vi "Pack for gRPC.vi"(8 "error in":errorcluster, 9 "configuration / results":enum16{"Configuration", "Results"}(ring), 10 "data value":variant, 11 "measurement plugin in":refnum<class "FPT_Compression.lvclass">) -> (0 "error out":errorcluster, 2 "any":T1, 3 "measurement plugin out":refnum<class "FPT_Compression.lvclass">)   [LabVIEW 2023, in "FPT_Compression.lvclass"]
uses:
  FPT_Compression.lvclass
  <vilib>/gRPC/LabVIEW gRPC Library/Shared/Any.ctl
  C:/Program Files/National Instruments/LabVIEW 2023/vi.lib/Plug-In SDKs/Measurements/Measurement Plugin Service/Measurement Plugin Service.lvclass
  Measurement Configuration.ctl
  Measurement Results.ctl
  2eca732d-dbaa-43bf-a7dd-ede2da65bc1b.vi
  a6012965-5700-4384-8228-972e71b6560c.vi
  <vilib>/gRPC/LabVIEW gRPC Library/Server API/Translate Protobuf Error.vi
  <vilib>/AdvancedString/1D String Array to Delimited String.vi
  <vilib>/gRPC/LabVIEW gRPC Library/Server API/Server/Get Server DLL Path.vi
  <vilib>/Plug-In SDKs/Measurements/Measurement Plugin Service/Measurement Plugin Service.lvclass
  <vilib>/gRPC/LabVIEW gRPC Library/grpc-lvsupport-release.lvlib
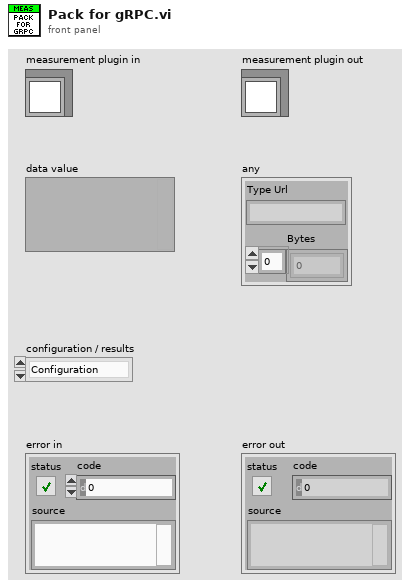
[diagram p1: front panel]
types:
  T1 = typedef "grpc-lvsupport-release.lvlib/Any.ctl" = cluster{"Type Url":string, "Bytes":u8[]}
  T2 = typedef "grpc-lvsupport-release.lvlib/grpcId.ctl" = u64
  T3 = typedef "FPT_Compression.lvclass/Measurement Configuration.ctl" = cluster{"Automation Test":bool, "Power sequencing file path":string, "SMU name":string, "SMU channel":string, "RFSG name":string, "RFSG port":string, "RFSG attenuation mode":enum32{"<None>", "Constant Attenuation", "s2p File"}, "RFSG external attenuation (dB)":dbl, "RFSG s-parameters orientation":enum32{"Port1 Towards DUT", "Port2 Towards DUT"}, "RFSG s2p file path":string, "RFmx name":string, "RFmx port":string, "RFmx attenuation mode":enum32{"<None>", "Constant Attenuation", "s2p File"}, "RFmx external attenuation (dB)":dbl, "RFmx attenuation path name":string, "RFmx s-parameters orientation":enum32{"Port1 Towards DUT", "Port2 Towards DUT"}, "RFmx attenuation s2p path name":string, "RFmx s2p file path":string, "Compression_Expected DUT Gain (dB)":dbl, "Compression_Max Linear Range (dBm)":dbl, "Compression_Compression Point (dB)":dbl, "Compression_Target Pin (dBm)":dbl, "Compression_RFSG Frequency Start (Hz)":dbl, "Compression_RFSG Frequency Stop (Hz)":dbl, "Compression_RFSG Number of Frequency Step":i32, "Compression_RFSG Power Start (dBm)":dbl, "Compression_RFSG Power Stop(dBm)":dbl, "Compression_RFSG Power Step Size (dB)":dbl, "Compression_RBW (Hz)":dbl, "Compression_RF Measurement Interval (s)":dbl, "Compression_DC Measurement Interval (s)":dbl, "Compression_Stimulus Mode":enum32{"Constant Power and RF", "Constant Power and Pulsed RF", "Pulsed Power and RF"}, "CP_CW_DC Source Delay (s)":dbl, "CP_PRF_DC Source Delay (s)":dbl, "CP_PRF_RFmx Trigger Delay (s)":dbl, "CP_PRF_RF Pulse Width (s)":dbl, "CP_PRF_PRI (s)":dbl, "PP_PRF_DC Source Delay (s)":dbl, "PP_PRF_RFmx Trigger Delay (s)":dbl, "PP_PRF_RF Pulse Width (s)":dbl, "PP_PRF_PRI (s)":dbl, "PP_PRF_DC Pulse Width (s)":dbl, "PP_PRF_ON Current Limit (A)":dbl, "PP_PRF_Bias Voltage Level (V)":dbl, "PP_PRF_Bias Current Limit (A)":dbl, "Power sequencing file validity check":bool}
  T4 = typedef "FPT_Compression.lvclass/Measurement Results.ctl" = cluster{"Status":string, "per Freq Plot Names":string[], "Linear Gain vs Freq":dbl[][], "OPxdB vs Freq":dbl[][], "Pout@Pin vs Freq":dbl[][], "Gain@Pin vs Freq":dbl[][], "PAE@Pin vs Freq":dbl[][], "Pout vs Pin per Freq":dbl[][], "Gain vs Pin per Freq":dbl[][], "PAE vs Pin per Freq":dbl[][], "Pout@Pin (Mean)":dbl, "Gain@Pin (Mean)":dbl, "PAE@Pin (Mean)":dbl, "Linear Gain (Mean)":dbl, "OPxdB (Mean)":dbl}
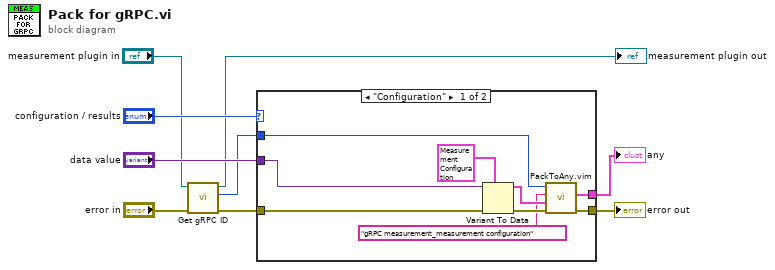
[diagram p0: block diagram]
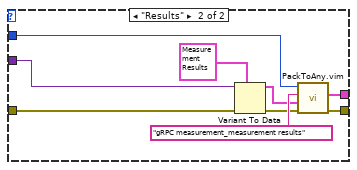
[diagram p2: hidden frame]
diagram:
  n1 = call <vilib>:"Get gRPC ID.vi"("error in"="error in", "measurement plugin service in"="measurement plugin in") -> ("error out"=w4:errorcluster, "gRPC ID"=w1:T2, "measurement plugin service out"=→"measurement plugin out":refnum<class "FPT_Compression.lvclass">)  [unwired: 7 in]
  n2 = case shown="\"Configuration\"" "configuration / results" {
    tunnel: w4 -> [w18 w27]
    tunnel: "data value" -> [w17 w26]
    tunnel: w1 -> [w14 w22]
    tunnel: [w16 w24] -> w8
    tunnel: [w15 w23] -> w7
    frame "Configuration" {
      n3 = Variant To Data(error in=w18, type=T3 {"Automation Test"=FALSE, "Power sequencing file path"="Lorem ipsum dolor sit", "SMU name"="", "SMU channel"="0", "RFSG name"="5842_0", "RFSG port"="", "RFSG attenuation mode"=enum."s2p File", "RFSG external attenuation (dB)"=64.0, "RFSG s-parameters orientation"=enum."Port1 Towards DUT", "RFSG s2p file path"="", "RFmx name"="Lorem ipsum dolor sit", "RFmx port"="", "RFmx attenuation mode"=enum."Constant Attenuation", "RFmx external attenuation (dB)"=-64.0, "RFmx attenuation path name"="", "RFmx s-parameters orientation"=enum."Port2 Towards DUT", "RFmx attenuation s2p path name"="", "RFmx s2p file path"="", "Compression_Expected DUT Gain (dB)"=17.5, "Compression_Max Linear Range (dBm)"=-10.0, "Compression_Compression Point (dB)"=1.0, "Compression_Target Pin (dBm)"=1.0, "Compression_RFSG Frequency Start (Hz)"=10000000000.0, "Compression_RFSG Frequency Stop (Hz)"=18000000000.0, "Compression_RFSG Number of Frequency Step"=10, "Compression_RFSG Power Start (dBm)"=-20.0, "Compression_RFSG Power Stop(dBm)"=1.0, "Compression_RFSG Power Step Size (dB)"=4.0, "Compression_RBW (Hz)"=0.0, "Compression_RF Measurement Interval (s)"=0.0, "Compression_DC Measurement Interval (s)"=0.001, "Compression_Stimulus Mode"=enum."Constant Power and RF", "CP_CW_DC Source Delay (s)"=0.0, "CP_PRF_DC Source Delay (s)"=0.0, "CP_PRF_RFmx Trigger Delay (s)"=0.0, "CP_PRF_RF Pulse Width (s)"=0.0001, "CP_PRF_PRI (s)"=0.001, "PP_PRF_DC Source Delay (s)"=0.0, "PP_PRF_RFmx Trigger Delay (s)"=0.0, "PP_PRF_RF Pulse Width (s)"=0.0001, "PP_PRF_PRI (s)"=0.001, "PP_PRF_DC Pulse Width (s)"=0.0008, "PP_PRF_ON Current Limit (A)"=2.0, "PP_PRF_Bias Voltage Level (V)"=0.0, "PP_PRF_Bias Current Limit (A)"=0.2, "Power sequencing file validity check"=FALSE} ("measurement configuration"), Variant=w17) -> (data=w13:T3, error out=w12:errorcluster)
      n4 = call "PackToAny.vim"("error in"=w12, "Data To Pack"=w13, "Message Type"="gRPC measurement_measurement configuration", "gRPCid in"=w14) -> ("error out"=w16:errorcluster, "Any"=w15:T1)  [unwired: 5 in, 1 out]
    }
    frame "Results" {
      n5 = Variant To Data(error in=w27, type=T4 {"Status"="Empty", "per Freq Plot Names"=[], "Linear Gain vs Freq"=[], "OPxdB vs Freq"=[], "Pout@Pin vs Freq"=[], "Gain@Pin vs Freq"=[], "PAE@Pin vs Freq"=[], "Pout vs Pin per Freq"=[], "Gain vs Pin per Freq"=[], "PAE vs Pin per Freq"=[], "Pout@Pin (Mean)"=0.0, "Gain@Pin (Mean)"=0.0, "PAE@Pin (Mean)"=0.0, "Linear Gain (Mean)"=0.0, "OPxdB (Mean)"=0.0} ("Measurement Results"), Variant=w26) -> (data=w20:T4, error out=w19:errorcluster)
      n6 = call "PackToAny.vim"("error in"=w19, "Data To Pack"=w20, "Message Type"="gRPC measurement_measurement results", "gRPCid in"=w22) -> ("error out"=w24:errorcluster, "Any"=w23:T1)  [unwired: 5 in, 1 out]
    }
  }
  "error out" <- w8
  "any" <- w7
